vi "SegmentedLineEdge_GetClassAttributesToModify.vi"(0 "reference in":refnum<class "SegmentedLineEdge.lvclass">, 3 "timeout (15000 ms)":i32=15000, 5 "error in (no error)":errorcluster) -> (14 "reference out":refnum<class "SegmentedLineEdge.lvclass">, 16 "Class attributes":T1, 17 "Timeout":bool, 19 "error out":errorcluster)   [LabVIEW 2012, in "SegmentedLineEdge.lvclass"]
doc: "This VI returns the class attributes associated with the object reference and places a lock on the object. If reference is wired, the class attributes of the class (or sub class) will be returned else the class attributes will default to the SegmentedLineEdge class.\n\nIf the object is currently locked for modification by another method, 'Timeout' specifies how long the VI should wait to receive access to the object. The default value waits until the object becomes available.\n\nYou must use the SegmentedLineEdge SetModifiedClassAttributes VI to set the object's data and release the lock.\n\n[GOOP 2.0.15]"
uses:
  <resource>/Framework/Providers/Open_GDS/UML/SegmentedLineEdge_class/SegmentedLineEdge.lvclass
  <resource>/Framework/Providers/Open_GDS/UML/SegmentedLineEdge_class/protected/ClassAttributes.ctl
  <resource>/Framework/Providers/Open_GDS/UML/GeneralPathEdge_class/protected/ClassAttributes.ctl
  <resource>/Framework/Providers/Open_GDS/UML/AbstractEdge_class/protected/ClassAttributes.ctl
  <resource>/Framework/Providers/Open_GDS/UML/SegmentedLineEdge_class/SegmentedLineEdge.lvclass/SegmentedLineEdge.ctl
  <vilib>/addons/_goop3.llb/3GOOPStates.ctl
  <resource>/Framework/Providers/Open_GDS/UML/AbstractEdge_class/AbstractEdge.lvclass
  <resource>/Framework/Providers/Open_GDS/UML/GeneralPathEdge_class/GeneralPathEdge.lvclass
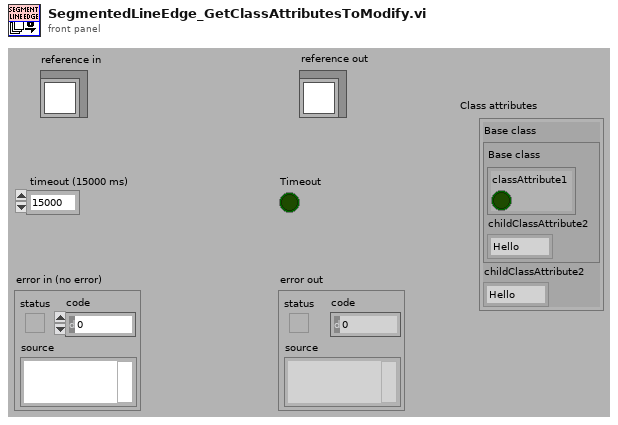
[diagram p1: front panel]
types:
  T1 = typedef "SegmentedLineEdge.lvclass/ClassAttributes.ctl" = cluster{"Base class":T2, "childClassAttribute2":enum16{"Hello", "Goodbye"}}
  T2 = typedef "GeneralPathEdge.lvclass/ClassAttributes.ctl" = cluster{"Base class":T3, "childClassAttribute2":enum16{"Hello", "Goodbye"}}
  T3 = typedef "AbstractEdge.lvclass/ClassAttributes.ctl" = cluster{"classAttribute1":bool}
  T4 = typedef "3GOOPStates.ctl" = enum16{"Set", "Get", "New", "Delete", "Clear", "Test and get", "Unlock data", "Information", "Look up existing", "New or look up existing", "Test and get shared", "Get shared", "Set shared", "Unlock shared", "Find dynamic method", "Register dynamic method", "Preload dynamic method", "Probe", "Cast to more generic", "Cast to more specific"}
  T5 = typedef "AbstractEdge.lvclass/ObjectReference.ctl" = refnum<k1>
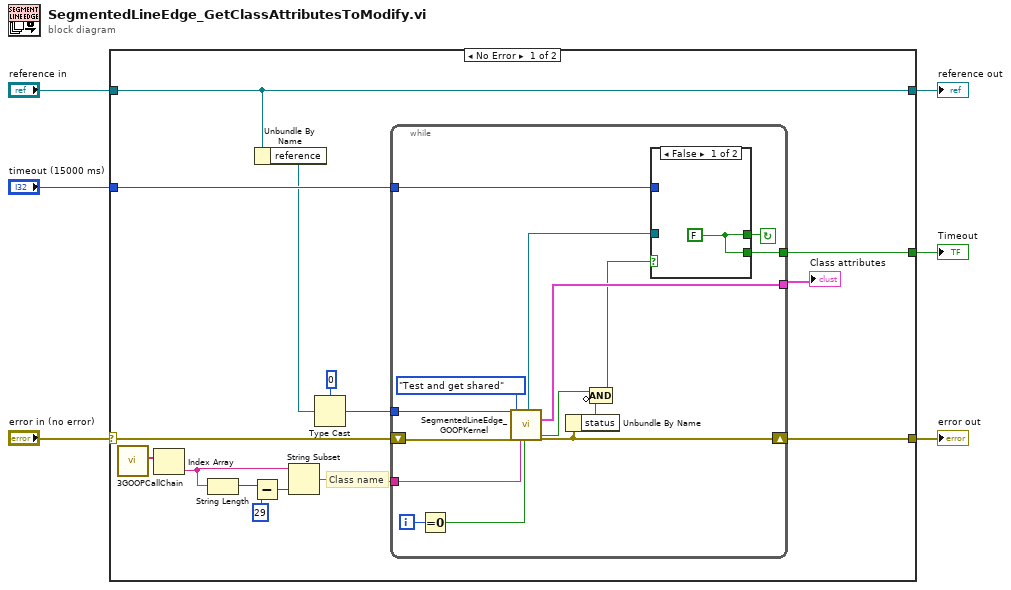
[diagram p0: block diagram]
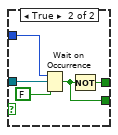
[diagram p2: hidden frame]
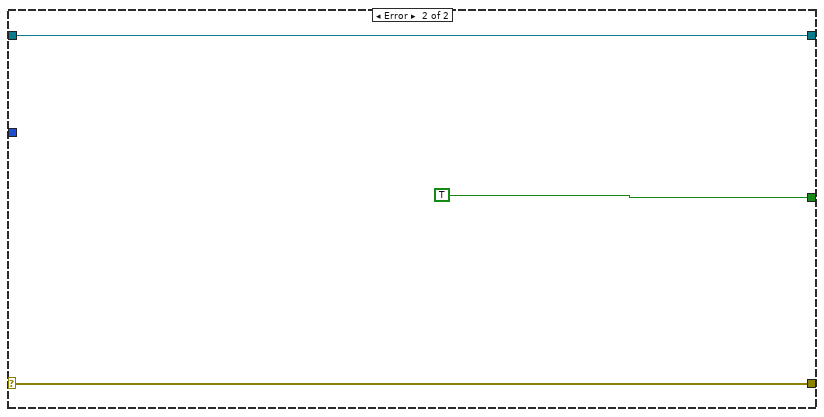
[diagram p3: hidden frame]
diagram:
  n1 = case shown="No Error" "error in (no error)" {
    selector: "error in (no error)" -> [w17 w44]
    tunnel: [w18 w45] -> w6
    tunnel: [w15 w44] -> w5
    tunnel: "reference in" -> [w18 w45]
    tunnel: "timeout (15000 ms)" -> [w21 _]
    tunnel: [w14 TRUE ("timed out")] -> w1
    frame No Error {
      # "Class name"
      n2 = call <vilib>:"3GOOPCallChain.vi"() -> ("call chain"=w7:string[])
      n3 = Index Array(array=w7) -> (element=w10:string)  [unwired: 1 in]
      n4 = String Length(string=w10) -> (length=w13:i32)
      n5 = Subtract(x=w13, y=29) -> (x-y=w11:i32)
      n6 = Unbundle By Name(w18) -> ("reference"=w8:T5)
      n7 = String Subset(string=w10, length (rest)=w11) -> (substring=w9:string)  [unwired: 1 out]
      n8 = Type Cast(type=0, x=w8) -> (*(type *) &x=w20:i32)
      n9 = while {
        tunnel: w9 -> [w22]
        tunnel: [w31] -> w16
        tunnel: w20 -> [w32]
        shift-left: w17 -> [w33]
        shift-right: [w29] -> w15
        tunnel: [w34] -> w14
        tunnel: w21 -> [w36]
        i -> [w26]
        stop <- w35 continue-if-true
        n10 = Equal To 0?(x=w26) -> (x = 0?=w25:bool)
        n11 = call <resource>:"SegmentedLineEdge_GOOPKernel.vi"("Ref in"=w32, "error in (no error)"=w33, "Action"=3GOOPStates."Test and get shared", "Dynamic VI name"=w22, "First try?"=w25) -> ("Occurrence out"=w24:refnum<k4>, "Data shared out"=w31:T1, "Data locked?"=w28:bool, "error out"=w29:errorcluster)  [unwired: 10 in, 9 out]
        n12 = Unbundle By Name(w29) -> ("status"=w30:bool)
        n13 = Compound Arithmetic op=AND(w28, invert w30) -> (w27:bool)
        n14 = case shown="False" w27 {
          tunnel: w24 -> [_ w41]
          tunnel: w36 -> [_ w42]
          tunnel: [w37 w39] -> w35
          tunnel: [w37 w38] -> w34
          frame False {
            w37 = FALSE
          }
          frame True {
            n15 = Wait on Occurrence(1:FALSE ("ignore previous (T)"), 2:w41, 3:w42) -> (0:w38:bool)
            n16 = Not(x=w38) -> (.not. x?=w39:bool)
          }
        }
      }
      "Class attributes" <- w16
    }
    frame Error {
    }
  }
  "error out" <- w5
  "reference out" <- w6
  "Timeout" <- w1
